vi "IOArray.vi"() -> ()   [LabVIEW 2015]
uses:
  <vilib>/Utility/file.llb/Read Delimited Spreadsheet (DBL).vi
  <vilib>/Utility/file.llb/Write Delimited Spreadsheet (DBL).vi
panel:
  out "first row":dbl[](array[numeric])
  out "all rows":dbl[][](array[numeric])=[[0.0, 0.0, 0.0, 0.0, 0.0, 0.0, 0.0, 0.0, 0.0, 0.0], [0.31, 0.803, 0.982, 0.699, 0.202, 0.373, 0.174, 0.243, 0.062, 0.433], [0.038, 0.897, 0.622, 0.74, 0.409, 1.598, 1.161, 1.716, 0.459, 1.455], [2.831, 1.969, 2.466, 1.386, 0.81, 1.999, 1.375, 1.862, 2.328, 0.528], [2.312, 2.967, 0.496, 3.682, 0.214, 3.945, 2.993, 0.601, 1.461, 2.583], [3.458, 0.129, 2.278, 0.206, 4.778, 1.735, 3.188, 0.421, 0.323, 0.438], [3.387, 0.01, 2.15, 1.785, 1.311, 1.943, 1.065, 1.17, 0.81, 5.634], [4.525, 3.473, 5.357, 2.374, 1.549, 0.682, 1.292, 6.574, 2.086, 6.126], [7.386, 4.667, 5.383, 4.347, 2.165, 4.948, 1.799, 7.195, 2.872, 4.331], [1.842, 6.14, 6.572, 6.469, 0.257, 7.206, 7.28, 8.205, 4.26, 3.218], [0.0, 0.0, 0.0, 0.0, 0.0, 0.0, 0.0, 0.0, 0.0, 0.0], [0.359, 0.109, 0.902, 0.952, 0.299, 0.464, 0.545, 0.907, 0.799, 0.02], [1.394, 0.961, 0.211, 1.28, 1.193, 1.724, 0.281, 1.337, 1.549, 0.674], [1.576, 2.356, 0.813, 1.581, 1.442, 1.628, 1.095, 2.983, 0.438, 1.083], [3.401, 3.639, 1.055, 3.5, 3.911, 1.51, 0.965, 1.313, 0.09, 0.043], [2.184, 4.74, 0.781, 2.545, 2.075, 1.509, 0.547, 3.108, 1.26, 1.307], [2.544, 2.729, 5.596, 5.277, 3.759, 4.902, 1.304, 3.974, 1.663, 3.362], [0.852, 0.41, 6.458, 4.943, 1.868, 2.112, 0.29, 1.344, 4.201, 5.265], [7.238, 4.912, 0.455, 7.248, 1.698, 6.716, 4.376, 4.101, 3.12, 6.502], [3.106, 0.547, 5.868, 0.833, 7.742, 4.487, 4.922, 2.065, 6.383, 5.071], [0.0, 0.448, 0.617, 0.075, 1.827, 2.199, 2.558, 1.742, 5.858, 2.206], [0.0, 0.123, 1.425, 1.025, 3.571, 3.792, 3.937, 4.75, 5.973, 6.031], [0.0, 0.83, 1.449, 2.919, 0.066, 2.676, 4.763, 2.837, 2.693, 3.224], [0.0, 0.257, 1.11, 0.712, 0.449, 1.933, 2.739, 5.732, 1.066, 6.829], [0.0, 0.421, 0.934, 2.324, 2.495, 2.17, 3.63, 1.833, 4.914, 1.165], [0.0, 0.468, 0.859, 1.189, 0.439, 2.285, 1.851, 6.501, 6.697, 6.474], [0.0, 0.583, 1.617, 0.055, 1.836, 2.352, 3.266, 3.014, 0.591, 8.926], [0.0, 0.565, 1.601, 0.219, 1.509, 4.765, 0.233, 0.275, 6.96, 0.85], [0.0, 0.27, 1.948, 0.866, 1.727, 2.53, 0.394, 6.505, 2.016, 5.348], [0.0, 0.136, 1.914, 1.447, 2.607, 3.501, 1.121, 6.153, 1.514, 5.808], [0.0, 0.6, 0.7, 0.5, 0.0, 4.7, 4.6, 4.5, 3.1, 7.3], [0.0, 0.2, 1.1, 2.4, 1.8, 2.4, 4.1, 6.8, 6.8, 6.3], [0.0, 0.5, 1.1, 1.8, 2.4, 3.3, 0.3, 2.6, 5.9, 2.4], [0.0, 0.4, 1.9, 0.9, 0.7, 3.3, 5.9, 4.5, 5.8, 7.4], [0.0, 0.2, 1.7, 2.5, 2.2, 2.1, 1.7, 2.5, 0.9, 0.9], [0.0, 0.9, 0.6, 2.3, 2.9, 0.3, 2.5, 3.7, 7.2, 3.0], [0.0, 0.2, 0.8, 2.3, 0.0, 4.5, 4.1, 3.7, 2.7, 5.1], [0.0, 1.0, 1.8, 2.5, 2.4, 2.4, 5.6, 6.5, 0.3, 7.8], [0.0, 0.8, 1.5, 1.3, 0.4, 0.6, 0.2, 4.4, 5.8, 1.8], [0.0, 0.7, 0.7, 0.1, 0.1, 4.0, 4.1, 2.2, 0.7, 3.9]]
  in  "Boolean":bool
  in  "file path (dialog if empty)":path=path "C:/Users/leser/Documents/LabVIEW Data/Apps/Lab Exercises/Prueba1.txt"
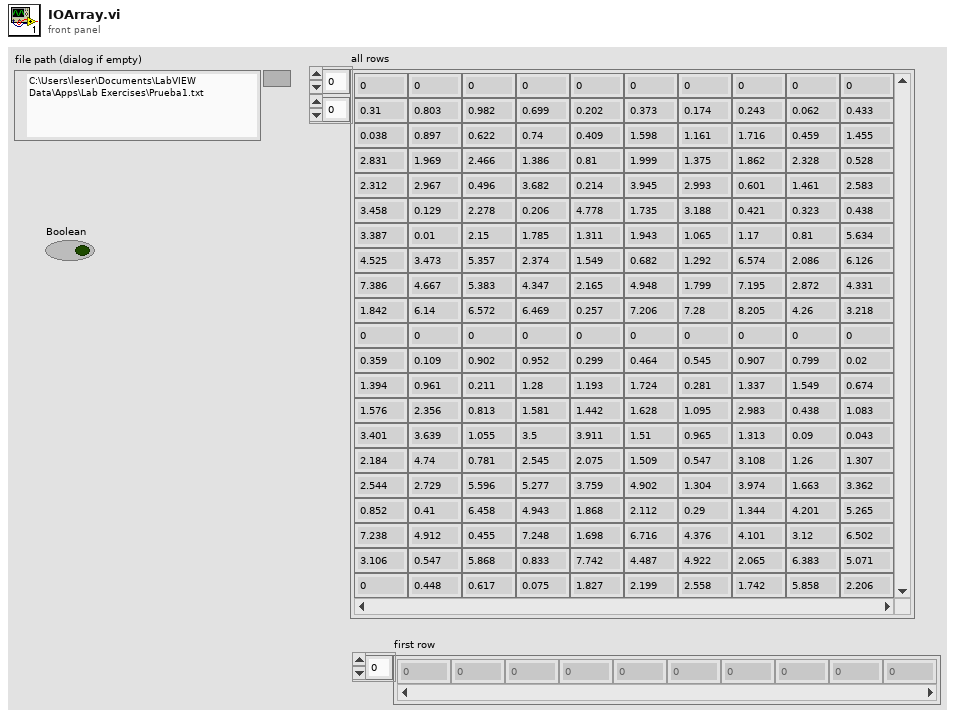
[diagram p1: front panel]
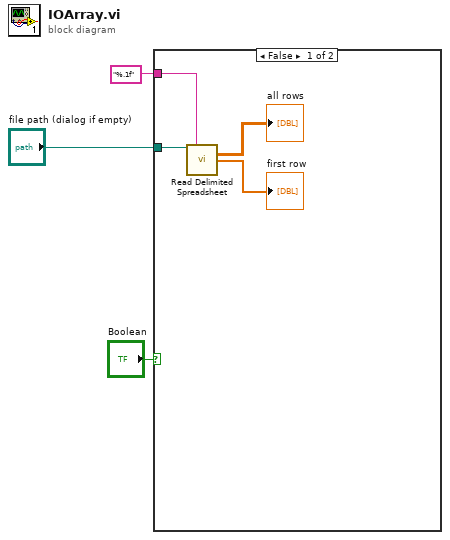
[diagram p0: block diagram]
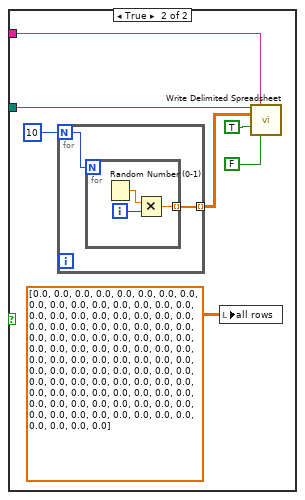
[diagram p2: hidden frame]
diagram:
  n1 = case shown="False" "Boolean" {
    tunnel: "%.1f" ("format (%.3f)") -> [w7 w10]
    tunnel: "file path (dialog if empty)" -> [w6 w9]
    frame False {
      n2 = call-poly <vilib>:"Read Delimited Spreadsheet.vi"("file path (dialog if empty)"=w6, "format (%.3f)"=w7) -> ("all rows"=→"all rows":dbl[][], "first row"=→"first row":dbl[])  [unwired: 8 in, 4 out]
    }
    frame True {
      n3 = for {
        N: 10 -> [w16]
        tunnel: [w15] -> w14 mode=indexing
        n4 = for {
          N: w16 -> [_]
          tunnel: [w17] -> w15 mode=indexing
          i -> [w18]
          n5 = Random Number (0-1)() -> (number: 0 to 1=w19:dbl)
          n6 = Multiply(x=w19, y=w18) -> (x*y=w17:dbl)
        }
      }
      n7 = local write "all rows"(dbl[][] [[0.0, 0.0, 0.0, 0.0, 0.0, 0.0, 0.0, 0.0, 0.0, 0.0], [0.0, 0.0, 0.0, 0.0, 0.0, 0.0, 0.0, 0.0, 0.0, 0.0], [0.0, 0.0, 0.0, 0.0, 0.0, 0.0, 0.0, 0.0, 0.0, 0.0], [0.0, 0.0, 0.0, 0.0, 0.0, 0.0, 0.0, 0.0, 0.0, 0.0], [0.0, 0.0, 0.0, 0.0, 0.0, 0.0, 0.0, 0.0, 0.0, 0.0], [0.0, 0.0, 0.0, 0.0, 0.0, 0.0, 0.0, 0.0, 0.0, 0.0], [0.0, 0.0, 0.0, 0.0, 0.0, 0.0, 0.0, 0.0, 0.0, 0.0], [0.0, 0.0, 0.0, 0.0, 0.0, 0.0, 0.0, 0.0, 0.0, 0.0], [0.0, 0.0, 0.0, 0.0, 0.0, 0.0, 0.0, 0.0, 0.0, 0.0], [0.0, 0.0, 0.0, 0.0, 0.0, 0.0, 0.0, 0.0, 0.0, 0.0]] ("all rows")) -> ()
      n8 = call-poly <vilib>:"Write Delimited Spreadsheet.vi"("file path (dialog if empty)"=w9, "format (%.3f)"=w10, "2D data"=w14, "append to file? (F)"=TRUE, "transpose? (F)"=FALSE) -> ()  [unwired: 9 in, 2 out]
    }
  }
